vi "Overlay Results (Matches).vi"(7 "Setup":T2, 8 "error in":errorcluster, 9 "Search Area":T1 {"Contours"."Type" items=["No Selection", "Point", "Line", "Rectangle", "Oval", "Polygon", "Free", "Annulus", "Unused2", "Unused3", "Broken Line", "Free Hand Line", "Rotated Rectangle"]}, 10 "Matches":T3(array[cluster]) {"Bounding Box"."y" format="%.2f"; "Bounding Box"."x" format="%.2f"; "Position"."y" format="%.2f"; "Position"."x" format="%.2f"; "Score" format="%.2f"; "Scale" format="%.2f"; "Angle" format="%.2f"}, 11 "Image In":T4) -> (0 "error out":errorcluster, 3 "Image Out":T4)   [LabVIEW 2018]
uses:
  <vilib>/vision/Image Controls.llb/IMAQ Image.ctl
panel:
  in  "Result Color":u32(colorbox)=16711680
  in  "Search Area Color":u32(colorbox)=65280
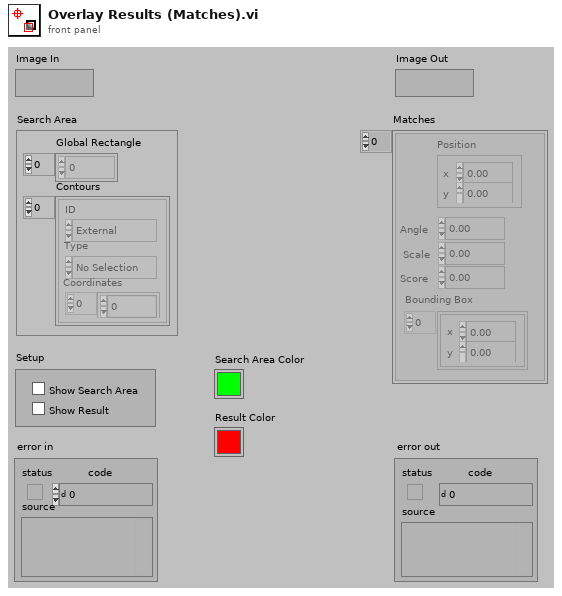
[diagram p1: front panel]
types:
  T1 = cluster{"Global Rectangle":i32[], "Contours":cluster{"ID":enum32{"External", "Internal"}, "Type":u32, "Coordinates":i32[]}[]}
  T2 = cluster{"Show Search Area":bool, "Show Result":bool}
  T3 = cluster{"Position":cluster{"x":sgl, "y":sgl}, "Angle":sgl, "Scale":sgl, "Score":sgl, "Bounding Box":cluster{"x":sgl, "y":sgl}[]}[]
  T4 = typedef "IMAQ Image.ctl" = refnum<image>
  T5 = cluster{"[0]":i32, "[1]":i32, "[2]":i32, "[3]":i32}
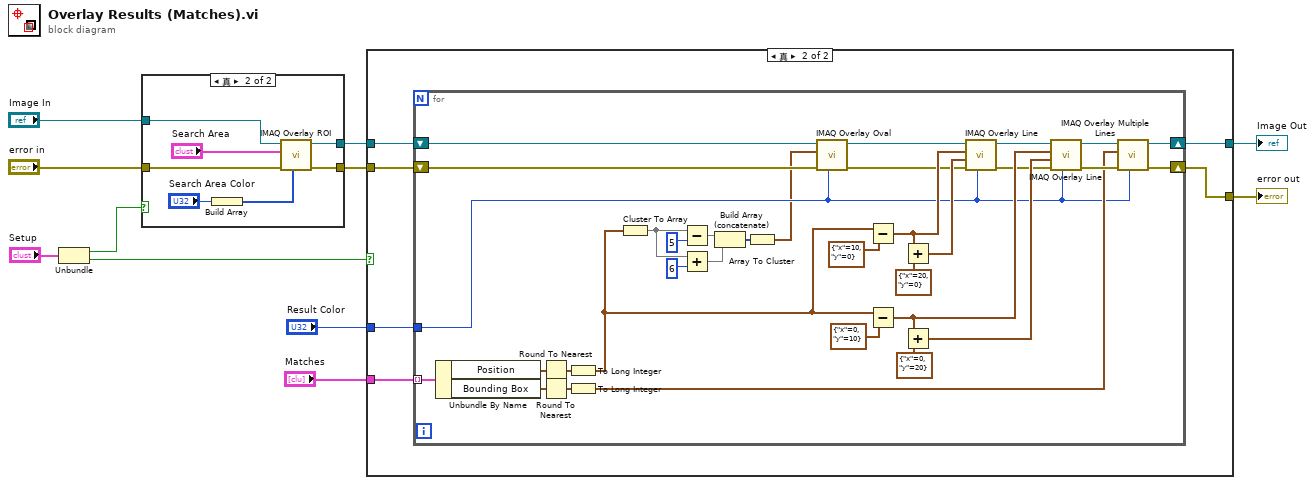
[diagram p0: block diagram]
diagram:
  n1 = Unbundle("Setup") -> ("Show Search Area"=w9:bool, "Show Result"=w7:bool)
  n2 = case shown="真" w9 {
    tunnel: "Image In" -> [w13 w20]
    tunnel: [w13 w19] -> w6
    tunnel: "error in" -> [w12 w16]
    tunnel: [w12 w15] -> w3
    frame False {
    }
    frame True {
      n3 = Build Array("Search Area Color") -> (w14:u32[])
      n4 = call "IMAQ Overlay ROI"("Colors (Green)"=w14, "error in (no error)"=w16, "ROI Descriptor"="Search Area", "Image"=w20) -> ("error out"=w15:errorcluster, "Image Out"=w19:T4)  [unwired: 2 in, 4 out]
    }
  }
  n5 = case shown="真" w7 {
    tunnel: w6 -> [w22 w28]
    tunnel: [w22 w26] -> w5
    tunnel: "Matches" -> [_ w27]
    tunnel: w3 -> [w21 w25]
    tunnel: [w21 w24] -> w2
    tunnel: "Result Color" -> [_ w23]
    frame False {
    }
    frame True {
      n6 = for {
        shift-right: [w60] -> w26
        shift-left: w28 -> [w61]
        tunnel: w27 -> [w58] mode=indexing
        shift-right: [w37] -> w24
        shift-left: w25 -> [w41]
        tunnel: w23 -> [w31]
        n7 = Unbundle By Name(w58) -> ("Position"=w36:cluster{"x":sgl, "y":sgl}, "Bounding Box"=w35:cluster{"x":sgl, "y":sgl}[])
        n8 = Round To Nearest(number=w36) -> (nearest integer value=w33:cluster{"x":sgl, "y":sgl})
        n9 = Round To Nearest(number=w35) -> (nearest integer value=w42:cluster{"x":sgl, "y":sgl}[])
        n10 = To Long Integer(number=w33) -> (32bit integer=w32:cluster{"x":i32, "y":i32})
        n11 = To Long Integer(number=w42) -> (32bit integer=w34:cluster{"x":i32, "y":i32}[])
        n12 = Cluster To Array(cluster=w32) -> (array=w29:i32[])
        n13 = Subtract(x=w29, y=5) -> (x-y=w56:i32[])
        n14 = Add(x=w29, y=6) -> (x+y=w55:i32[])
        n15 = Build Array (concatenate)(w56, w55) -> (w52:i32[])
        n16 = Array To Cluster(array=w52) -> (cluster=w30:T5)
        n17 = call "IMAQ Overlay Oval"("Color"=w31, "error in (no error)"=w41, "Bounding Rectangle"=w30, "Image"=w61) -> ("error out"=w40:errorcluster, "Image Out"=w59:T4)  [unwired: 2 in, 4 out]
        n18 = Subtract(x=w32, y=cluster{"x":i32, "y":i32} {"x"=10, "y"=0}) -> (x-y=w48:cluster{"x":i32, "y":i32})
        n19 = Subtract(x=w32, y=cluster{"x":i32, "y":i32} {"x"=0, "y"=10}) -> (x-y=w47:cluster{"x":i32, "y":i32})
        n20 = Add(x=w48, y=cluster{"x":i32, "y":i32} {"x"=20, "y"=0}) -> (x+y=w49:cluster{"x":i32, "y":i32})
        n21 = Add(x=w47, y=cluster{"x":i32, "y":i32} {"x"=0, "y"=20}) -> (x+y=w46:cluster{"x":i32, "y":i32})
        n22 = call "IMAQ Overlay Line"("Color"=w31, "error in (no error)"=w40, "End Point"=w49, "Start Point"=w48, "Image"=w59) -> ("error out"=w39:errorcluster, "Image Out"=w43:T4)  [unwired: 1 in, 4 out]
        n23 = call "IMAQ Overlay Line"("Color"=w31, "error in (no error)"=w39, "End Point"=w46, "Start Point"=w47, "Image"=w43) -> ("error out"=w38:errorcluster, "Image Out"=w57:T4)  [unwired: 1 in, 4 out]
        n24 = call "IMAQ Overlay Multiple Lines"("Color"=w31, "error in (no error)"=w38, "Line End Points"=w34, "Image"=w57) -> ("error out"=w37:errorcluster, "Image Out"=w60:T4)  [unwired: 2 in, 4 out]
      }
    }
  }
  "error out" <- w2
  "Image Out" <- w5
